vi "UHR-Fleezers Control (host) - Lorentz v3.vi"() -> ()   [LabVIEW 2014] (continued)
            n1765 = Number To Decimal String(number=w2676) -> (decimal integer string=w2678:string)  [unwired: 1 in]
            n1766 = Concatenate Strings("on, flow rate", w2678) -> (w2677:string)
            n1767 = Select(t=w2677, s=w2682, f="off") -> (s? t:f=w2686:string)
            n1768 = local read "Time (s)"() -> (w2680:dbl)
            n1769 = local read "log file ref"() -> (w2681:refnum<file>)
            n1770 = Concatenate Strings("pump 2 ", w2686) -> (w2684:string)
            n1771 = call "write to event log.vi"("log file ref"=w2681, "time"=w2680, "input string"=w2684) -> ()  [unwired: 8 in]
          }
        }
      }
      event "Sample Channel\nFlow": Value Change {
        n1772 = event-data() -> ()  [unwired: 7 out]
        n1773 = disable-structure shown="Disabled" {
          disable-tunnel: w2704 -> [w2711 _]
          frame Disabled {
            n1774 = Select(t="irun" ("string"), s="Sample Channel\nFlow", f="stop" ("string")) -> (s? t:f=w2706:string)
            n1775 = Concatenate Strings(w2706, "\r") -> (w2709:string)
            n1776 = VISA Write(VISA resource name=w2711, write buffer=w2709) -> ()  [unwired: 1 in, 3 out]
          }
          frame Enabled {
          }
        }
      }
      event "Start Flow": Value Change {
        n1777 = event-data() -> ()  [unwired: 7 out]
        n1778 = disable-structure shown="Disabled" {
          disable-tunnel: w2712 -> [w2713 _]
          frame Disabled {
            n1779 = local write "Sample Channel\nFlow"(TRUE ("Sample Channel\nFlow")) -> ()
            n1780 = local write "Start Flow"(FALSE ("Start Flow")) -> ()
            n1781 = Concatenate Strings("irun" ("string"), "\r") -> (w2717:string)
            n1782 = VISA Write(VISA resource name=w2713, write buffer=w2717) -> ()  [unwired: 1 in, 3 out]
          }
          frame Enabled {
          }
        }
      }
      event "Stop Flow": Value Change {
        n1783 = event-data() -> ()  [unwired: 7 out]
        n1784 = disable-structure shown="Disabled" {
          disable-tunnel: w2719 -> [w2721 _]
          frame Disabled {
            w2720 = FALSE ("Stop Flow")
            n1785 = local write "Stop Flow"(w2720) -> ()
            n1786 = local write "Sample Channel\nFlow"(w2720) -> ()
            n1787 = Concatenate Strings("stop" ("string"), "\r") -> (w2723:string)
            n1788 = VISA Write(VISA resource name=w2721, write buffer=w2723) -> ()  [unwired: 1 in, 3 out]
          }
          frame Enabled {
          }
        }
      }
      event "Flow rate (uL/h)": Value Change {
        n1789 = event-data() -> ()  [unwired: 7 out]
        n1790 = disable-structure shown="Disabled" {
          disable-tunnel: w2725 -> [w2727 _]
          frame Disabled {
            n1791 = Number To Decimal String(number="Flow rate (uL/h)") -> (decimal integer string=w2731:string)  [unwired: 1 in]
            n1792 = Concatenate Strings("irate  " ("string"), w2731, " u/h" ("string"), "\r") -> (w2730:string)
            n1793 = VISA Write(VISA resource name=w2727, write buffer=w2730) -> ()  [unwired: 1 in, 3 out]
          }
          frame Enabled {
          }
        }
      }
      event "Flush Sample": Value Change {
        n1794 = event-data() -> ()  [unwired: 7 out]
        n1795 = disable-structure shown="Disabled" {
          disable-tunnel: ["Flush Sample" _] -> w2734
          disable-tunnel: w2733 -> [w2740 _]
          frame Disabled {
            n1796 = flat-sequence {
              tunnel: w2740 -> [w2781]
              tunnel: [w2761] -> w2744
              tunnel: [w2757] -> w2743
              tunnel: ["Volume (uL)"] -> w2739
              tunnel: ["Flush rate (uL/m)"] -> w2738
              tunnel: w2744 -> [w2785]
              tunnel: [w2785] -> w2742
              tunnel: w2743 -> [w2784]
              tunnel: w2742 -> [w2790]
              frame #0 {
                # "set paramaters (rate, volume) for flush, clear volume"
                n1797 = Number To Decimal String(number="Flush rate (uL/m)") -> (decimal integer string=w2777:string)  [unwired: 1 in]
                n1798 = Concatenate Strings("irate  " ("string"), w2777, " u/m" ("string"), "\r") -> (w2779:string)
                n1799 = VISA Write(VISA resource name=w2781, write buffer=w2779) -> (VISA resource name out=w2775:refnum<visa-resource-name>)  [unwired: 1 in, 2 out]
                n1800 = Reciprocal(x="Flush rate (uL/m)") -> (1/x=w2760:dbl)
                n1801 = Number To Decimal String(number="Volume (uL)") -> (decimal integer string=w2766:string)  [unwired: 1 in]
                n1802 = Multiply(x="Volume (uL)", y=w2760) -> (x*y=w2759:dbl)
                n1803 = Concatenate Strings("tvolume  " ("string"), w2766, " u" ("string"), "\r") -> (w2764:string)
                n1804 = Multiply(x=w2759, y=60000.0) -> (x*y=w2757:dbl)
                n1805 = VISA Write(VISA resource name=w2775, write buffer=w2764) -> (VISA resource name out=w2763:refnum<visa-resource-name>)  [unwired: 1 in, 2 out]
                n1806 = Concatenate Strings("cvolume" ("string"), "\r") -> (w2762:string)
                n1807 = VISA Write(VISA resource name=w2763, write buffer=w2762) -> (VISA resource name out=w2773:refnum<visa-resource-name>)  [unwired: 1 in, 2 out]
                n1808 = Concatenate Strings("irun" ("string"), "\r") -> (w2771:string)
                n1809 = VISA Write(VISA resource name=w2773, write buffer=w2771) -> (VISA resource name out=w2761:refnum<visa-resource-name>)  [unwired: 1 in, 2 out]
              }
              frame #1 {
                # "Have to wait until\nflow is done to reset\nrate"
                n1810 = Add(x=w2784, y=100.0) -> (x+y=w2783:dbl)
                n1811 = Wait (ms)(milliseconds to wait=w2783) -> ()  [unwired: 1 out]
              }
              frame #2 {
                # "reset flow rate to usual flow rate"
                n1812 = local read "Flow rate (uL/h)"() -> (w2796:dbl)
                n1813 = Number To Decimal String(number=w2796) -> (decimal integer string=w2794:string)  [unwired: 1 in]
                n1814 = Concatenate Strings("irate  " ("string"), w2794, " u/h" ("string"), "\r") -> (w2792:string)
                n1815 = VISA Write(VISA resource name=w2790, write buffer=w2792) -> (VISA resource name out=w2786:refnum<visa-resource-name>)  [unwired: 1 in, 2 out]
                n1816 = Concatenate Strings("cvolume" ("string"), "\r") -> (w2787:string)
                n1817 = VISA Write(VISA resource name=w2786, write buffer=w2787) -> ()  [unwired: 1 in, 3 out]
              }
            }
            n1818 = local read "Save Event Log?"() -> (w2736:bool)
            n1819 = local read "Saving..."() -> (w2735:bool)
            n1820 = And(x=w2736, y=w2735) -> (x .and. y?=w2737:bool)
            n1821 = case shown="True" w2737 {
              tunnel: w2739 -> [_ w2746]
              tunnel: w2738 -> [_ w2745]
              frame False {
              }
              frame True {
                n1822 = Number To Decimal String(number=w2746) -> (decimal integer string=w2750:string)  [unwired: 1 in]
                n1823 = Number To Decimal String(number=w2745) -> (decimal integer string=w2752:string)  [unwired: 1 in]
                n1824 = local read "log file ref"() -> (w2747:refnum<file>)
                n1825 = local read "Time (s)"() -> (w2748:dbl)
                n1826 = Concatenate Strings("pump 2 flushing ", w2750, " uL at ", w2752, " ul/min") -> (w2754:string)
                n1827 = call "write to event log.vi"("log file ref"=w2747, "time"=w2748, "input string"=w2754) -> ()  [unwired: 8 in]
              }
            }
          }
          frame Enabled {
          }
        }
      }
      event "Flush Pump 3": Value Change {
        n1828 = event-data() -> ()  [unwired: 7 out]
        n1829 = disable-structure shown="Disabled" {
          disable-tunnel: ["Flush Pump 3" _] -> w2798
          disable-tunnel: w2797 -> [w2804 _]
          frame Disabled {
            n1830 = flat-sequence {
              tunnel: w2804 -> [w2819]
              tunnel: ["Flush rate (uL/m) P3"] -> w2800
              tunnel: ["Volume (uL) P3"] -> w2799
              frame #0 {
                # "set paramaters (rate, volume) for flush, clear volume"
                n1831 = Number To Decimal String(number="Flush rate (uL/m) P3") -> (decimal integer string=w2839:string)  [unwired: 1 in]
                n1832 = local write "Inject Pump 3"(TRUE ("Inject Pump 3")) -> ()
                n1833 = Concatenate Strings("irate  " ("string"), w2839, " u/m" ("string"), "\r") -> (w2841:string)
                n1834 = VISA Write(VISA resource name=w2819, write buffer=w2841) -> (VISA resource name out=w2837:refnum<visa-resource-name>)  [unwired: 1 in, 2 out]
                n1835 = Reciprocal(x="Flush rate (uL/m) P3") -> (1/x=w2823:dbl)
                n1836 = Number To Decimal String(number="Volume (uL) P3") -> (decimal integer string=w2828:string)  [unwired: 1 in]
                n1837 = Multiply(x="Volume (uL) P3", y=w2823) -> (x*y=w2822:dbl)
                n1838 = Concatenate Strings("tvolume  " ("string"), w2828, " u" ("string"), "\r") -> (w2826:string)
                n1839 = Multiply(x=w2822, y=60.0) -> (x*y=→"HP3 Flush Time (s)":dbl)
                n1840 = VISA Write(VISA resource name=w2837, write buffer=w2826) -> (VISA resource name out=w2825:refnum<visa-resource-name>)  [unwired: 1 in, 2 out]
                n1841 = Concatenate Strings("cvolume" ("string"), "\r") -> (w2824:string)
                n1842 = VISA Write(VISA resource name=w2825, write buffer=w2824) -> (VISA resource name out=w2835:refnum<visa-resource-name>)  [unwired: 1 in, 2 out]
                n1843 = Concatenate Strings("irun" ("string"), "\r") -> (w2833:string)
                n1844 = VISA Write(VISA resource name=w2835, write buffer=w2833) -> ()  [unwired: 1 in, 3 out]
              }
              frame #1 {
                "Flushing P3" <- TRUE ("Flushing P3")
              }
            }
            n1845 = local read "Save Event Log?"() -> (w2802:bool)
            n1846 = local read "Saving..."() -> (w2803:bool)
            n1847 = And(x=w2802, y=w2803) -> (x .and. y?=w2801:bool)
            n1848 = case shown="True" w2801 {
              tunnel: w2800 -> [_ w2807]
              tunnel: w2799 -> [_ w2806]
              frame False {
              }
              frame True {
                n1849 = Number To Decimal String(number=w2806) -> (decimal integer string=w2811:string)  [unwired: 1 in]
                n1850 = Number To Decimal String(number=w2807) -> (decimal integer string=w2813:string)  [unwired: 1 in]
                n1851 = local read "log file ref"() -> (w2808:refnum<file>)
                n1852 = local read "Time (s)"() -> (w2809:dbl)
                n1853 = Concatenate Strings("pump 3 flushing ", w2811, " uL at ", w2813, " ul/min") -> (w2815:string)
                n1854 = call "write to event log.vi"("log file ref"=w2808, "time"=w2809, "input string"=w2815) -> ()  [unwired: 8 in]
              }
            }
          }
          frame Enabled {
          }
        }
      }
      event "Flush Pump 1": Value Change {
        n1855 = event-data() -> ()  [unwired: 7 out]
        n1856 = disable-structure shown="Disabled" {
          disable-tunnel: ["Flush Pump 1" _] -> w2845
          disable-tunnel: w2844 -> [w2851 _]
          frame Disabled {
            n1857 = flat-sequence {
              tunnel: [w2872] -> w2853
              tunnel: w2851 -> [w2867]
              tunnel: ["Volume (uL) P1"] -> w2847
              tunnel: ["Flush rate (uL/m) P1"] -> w2846
              tunnel: w2853 -> [_]
              frame #0 {
                # "set paramaters (rate, volume) for flush, clear volume"
                n1858 = local write "Inject Pump 1"(TRUE ("Inject Pump 1")) -> ()
                n1859 = Number To Decimal String(number="Flush rate (uL/m) P1") -> (decimal integer string=w2888:string)  [unwired: 1 in]
                n1860 = Concatenate Strings("irate  " ("string"), w2888, " u/m" ("string"), "\r") -> (w2890:string)
                n1861 = VISA Write(VISA resource name=w2867, write buffer=w2890) -> (VISA resource name out=w2886:refnum<visa-resource-name>)  [unwired: 1 in, 2 out]
                n1862 = Reciprocal(x="Flush rate (uL/m) P1") -> (1/x=w2871:dbl)
                n1863 = Number To Decimal String(number="Volume (uL) P1") -> (decimal integer string=w2877:string)  [unwired: 1 in]
                n1864 = Multiply(x="Volume (uL) P1", y=w2871) -> (x*y=w2870:dbl)
                n1865 = Concatenate Strings("tvolume  " ("string"), w2877, " u" ("string"), "\r") -> (w2875:string)
                n1866 = Multiply(x=w2870, y=60.0) -> (x*y=→"HP1 Flush Time (s)":dbl)
                n1867 = VISA Write(VISA resource name=w2886, write buffer=w2875) -> (VISA resource name out=w2874:refnum<visa-resource-name>)  [unwired: 1 in, 2 out]
                n1868 = Concatenate Strings("cvolume" ("string"), "\r") -> (w2873:string)
                n1869 = VISA Write(VISA resource name=w2874, write buffer=w2873) -> (VISA resource name out=w2884:refnum<visa-resource-name>)  [unwired: 1 in, 2 out]
                n1870 = Concatenate Strings("irun" ("string"), "\r") -> (w2882:string)
                n1871 = VISA Write(VISA resource name=w2884, write buffer=w2882) -> (VISA resource name out=w2872:refnum<visa-resource-name>)  [unwired: 1 in, 2 out]
              }
              frame #1 {
                "Flushing P1" <- TRUE ("Flushing P3")
              }
            }
            n1872 = local read "Saving..."() -> (w2848:bool)
            n1873 = local read "Save Event Log?"() -> (w2849:bool)
            n1874 = And(x=w2849, y=w2848) -> (x .and. y?=w2850:bool)
            n1875 = case shown="True" w2850 {
              tunnel: w2847 -> [_ w2856]
              tunnel: w2846 -> [_ w2855]
              frame False {
              }
              frame True {
                n1876 = Number To Decimal String(number=w2856) -> (decimal integer string=w2860:string)  [unwired: 1 in]
                n1877 = Number To Decimal String(number=w2855) -> (decimal integer string=w2858:string)  [unwired: 1 in]
                n1878 = local read "log file ref"() -> (w2862:refnum<file>)
                n1879 = local read "Time (s)"() -> (w2863:dbl)
                n1880 = Concatenate Strings("pump 1 flushing ", w2860, " uL at ", w2858, " ul/min") -> (w2854:string)
                n1881 = call "write to event log.vi"("log file ref"=w2862, "time"=w2863, "input string"=w2854) -> ()  [unwired: 8 in]
              }
            }
          }
          frame Enabled {
          }
        }
      }
      event "Clear Volume": Value Change {
        n1882 = event-data() -> ()  [unwired: 7 out]
        n1883 = disable-structure shown="Disabled" {
          disable-tunnel: ["Clear Volume" _] -> w2894
          disable-tunnel: w2893 -> [w2895 _]
          frame Disabled {
            n1884 = Concatenate Strings("cvolume" ("string"), "\r") -> (w2896:string)
            n1885 = VISA Write(VISA resource name=w2895, write buffer=w2896) -> ()  [unwired: 1 in, 3 out]
          }
          frame Enabled {
          }
        }
      }
      event "Clear Volume P3": Value Change {
        n1886 = event-data() -> ()  [unwired: 7 out]
        n1887 = disable-structure shown="Disabled" {
          disable-tunnel: w2900 -> [w2902 _]
          frame Disabled {
            n1888 = Concatenate Strings("cvolume" ("string"), "\r") -> (w2903:string)
            n1889 = VISA Write(VISA resource name=w2902, write buffer=w2903) -> ()  [unwired: 1 in, 3 out]
            n1890 = local write "Clear Volume P3"(FALSE ("Clear Volume P3")) -> ()
          }
          frame Enabled {
          }
        }
      }
      event "Clear Volume P1": Value Change {
        n1891 = event-data() -> ()  [unwired: 7 out]
        n1892 = disable-structure shown="Disabled" {
          disable-tunnel: w2906 -> [w2908 _]
          frame Disabled {
            n1893 = Concatenate Strings("cvolume" ("string"), "\r") -> (w2909:string)
            n1894 = local write "Clear Volume P1"(FALSE ("Clear Volume P1")) -> ()
            n1895 = VISA Write(VISA resource name=w2908, write buffer=w2909) -> ()  [unwired: 1 in, 3 out]
          }
          frame Enabled {
          }
        }
      }
      event "Display On P3": Value Change {
        n1896 = event-data() -> ()  [unwired: 7 out]
        n1897 = disable-structure shown="Disabled" {
          disable-tunnel: w2912 -> [w2913 _]
          frame Disabled {
            n1898 = Select(t="dim 100", s="Display On P3", f="dim 0") -> (s? t:f=w2916:string)
            n1899 = Concatenate Strings(w2916, "\r") -> (w2918:string)
            n1900 = VISA Write(VISA resource name=w2913, write buffer=w2918) -> ()  [unwired: 1 in, 3 out]
          }
          frame Enabled {
          }
        }
      }
      event "Display On P1": Value Change {
        n1901 = event-data() -> ()  [unwired: 7 out]
        n1902 = disable-structure shown="Disabled" {
          disable-tunnel: w2920 -> [w2921 _]
          frame Disabled {
            n1903 = Select(t="dim 100", s="Display On P1", f="dim 0") -> (s? t:f=w2924:string)
            n1904 = Concatenate Strings(w2924, "\r") -> (w2926:string)
            n1905 = VISA Write(VISA resource name=w2921, write buffer=w2926) -> ()  [unwired: 1 in, 3 out]
          }
          frame Enabled {
          }
        }
      }
      event "Retract Pump 3": Value Change {
        n1906 = event-data() -> ()  [unwired: 7 out]
        n1907 = disable-structure shown="Disabled" {
          disable-tunnel: w2928 -> [w2929 _]
          frame Disabled {
            n1908 = local write "Retract Pump 3"(FALSE ("Retract Pump 3")) -> ()
            n1909 = case shown="True" "Retract Pump 3" {
              tunnel: w2929 -> [_ w2932]
              frame False {
              }
              frame True {
                n1910 = Number To Decimal String(number="Retract Rate (uL/m)") -> (decimal integer string=w2950:string)  [unwired: 1 in]
                n1911 = Concatenate Strings("wrate  " ("string"), w2950, " u/m" ("string"), "\r") -> (w2952:string)
                n1912 = VISA Write(VISA resource name=w2932, write buffer=w2952) -> (VISA resource name out=w2943:refnum<visa-resource-name>)  [unwired: 1 in, 2 out]
                n1913 = Number To Decimal String(number="Retract Vol 3 (uL)") -> (decimal integer string=w2945:string)  [unwired: 1 in]
                n1914 = Concatenate Strings("tvolume  " ("string"), w2945, " u" ("string"), "\r") -> (w2942:string)
                n1915 = VISA Write(VISA resource name=w2943, write buffer=w2942) -> (VISA resource name out=w2938:refnum<visa-resource-name>)  [unwired: 1 in, 2 out]
                n1916 = Concatenate Strings("cvolume" ("string"), "\r") -> (w2939:string)
                n1917 = VISA Write(VISA resource name=w2938, write buffer=w2939) -> (VISA resource name out=w2933:refnum<visa-resource-name>)  [unwired: 1 in, 2 out]
                n1918 = Concatenate Strings("wrun" ("string"), "\r") -> (w2934:string)
                n1919 = VISA Write(VISA resource name=w2933, write buffer=w2934) -> ()  [unwired: 1 in, 3 out]
              }
            }
          }
          frame Enabled {
          }
        }
      }
      event "Retract Pump 1": Value Change {
        n1920 = event-data() -> ()  [unwired: 7 out]
        n1921 = disable-structure shown="Disabled" {
          disable-tunnel: w2954 -> [w2955 _]
          frame Disabled {
            n1922 = local write "Retract Pump 1"(FALSE ("Retract Pump 1")) -> ()
            n1923 = case shown="True" "Retract Pump 1" {
              tunnel: w2955 -> [_ w2960]
              frame False {
              }
              frame True {
                n1924 = local read "Retract Rate (uL/m)"() -> (w2958:dbl)
                n1925 = Number To Decimal String(number=w2958) -> (decimal integer string=w2976:string)  [unwired: 1 in]
                n1926 = Concatenate Strings("wrate  " ("string"), w2976, " u/m" ("string"), "\r") -> (w2978:string)
                n1927 = VISA Write(VISA resource name=w2960, write buffer=w2978) -> (VISA resource name out=w2970:refnum<visa-resource-name>)  [unwired: 1 in, 2 out]
                n1928 = Number To Decimal String(number="Retract Vol 1 (uL)") -> (decimal integer string=w2972:string)  [unwired: 1 in]
                n1929 = Concatenate Strings("tvolume  " ("string"), w2972, " u" ("string"), "\r") -> (w2969:string)
                n1930 = VISA Write(VISA resource name=w2970, write buffer=w2969) -> (VISA resource name out=w2966:refnum<visa-resource-name>)  [unwired: 1 in, 2 out]
                n1931 = Concatenate Strings("cvolume" ("string"), "\r") -> (w2967:string)
                n1932 = VISA Write(VISA resource name=w2966, write buffer=w2967) -> (VISA resource name out=w2961:refnum<visa-resource-name>)  [unwired: 1 in, 2 out]
                n1933 = Concatenate Strings("wrun" ("string"), "\r") -> (w2962:string)
                n1934 = VISA Write(VISA resource name=w2961, write buffer=w2962) -> ()  [unwired: 1 in, 3 out]
              }
            }
          }
          frame Enabled {
          }
        }
      }
      event "Flip Green Filter": Value Change {
        n1935 = event-data() -> ()  [unwired: 7 out]
        n1936 = Not(x="Flip Green Filter") -> (.not. x?=w2981:bool)
        n1937 = local write "Flip Green Filter"(w2981) -> ()
        n1938 = flat-sequence {
          tunnel: [w2990] -> w2986
          tunnel: [w2989] -> w2985
          tunnel: w2980 -> [w2988]
          tunnel: [w2993] -> w2984
          tunnel: w2986 -> [w2993]
          tunnel: [w2992] -> w2983
          tunnel: w2985 -> [w2992]
          tunnel: w2984 -> [w2997]
          tunnel: w2983 -> [w2996]
          tunnel: [w2995] -> w2987
          frame #0 {
            n1939 = xnode "Read/Write Control"("FPGA VI Reference In"=w2988, "Green Filter Flipper"=TRUE) -> ("FPGA VI Reference Out"=w2990:T36, "error out"=w2989:errorcluster)  [unwired: 1 in]
          }
          frame #1 {
            n1940 = Wait (ms)(milliseconds to wait=u32 100) -> ()  [unwired: 1 out]
          }
          frame #2 {
            n1941 = xnode "Read/Write Control"("FPGA VI Reference In"=w2997, "error in"=w2996, "Green Filter Flipper"=FALSE) -> ("error out"=w2995:errorcluster)  [unwired: 1 out]
          }
        }
      }
      event "Pump 1 contents", "Pump 3 contents": Value Change {
        n1942 = event-data() -> ()  [unwired: 7 out]
        n1943 = local read "Pump 1 contents"() -> (→"Pump 1 cont disp":string)
        n1944 = local read "Pump 3 contents"() -> (→"Pump 3 cont disp":string)
      }
      event "Reset Trap Pos. FB": Value Change {
        n1945 = event-data() -> ()  [unwired: 7 out]
        n1946 = xnode "Read/Write Control"("FPGA VI Reference In"=w3001, "Trap Pos. FB Reset"="Reset Trap Pos. FB") -> ()  [unwired: 1 in, 2 out]
      }
      event "Rem fb disp offset": Value Change {
        n1947 = event-data() -> ()  [unwired: 7 out]
        n1948 = local write "Rem fb disp offset"(FALSE ("Rem fb disp offset")) -> ()
        n1949 = local read "Mean Trap Positions (nm)"() -> (w3004:T4)
        n1950 = local read "FB Trap Pos Offset"() -> (w3006:dbl)
        n1951 = Unbundle By Name(w3004) -> ("T1 X"=w3003:dbl)
        n1952 = Subtract(x=w3006, y=w3003) -> (x-y=w3005:dbl)
        n1953 = local write "FB Trap Pos Offset"(w3005) -> ()
      }
      event "Threshold (nm)": Value Change {
        n1954 = event-data() -> ()  [unwired: 7 out]
        n1955 = flat-sequence {
          tunnel: [w3011] -> w3009
          tunnel: w3008 -> [w3010]
          tunnel: w3009 -> [w3022]
          frame #0 {
            n1956 = xnode "Read/Write Control"("FPGA VI Reference In"=w3010) -> ("FPGA VI Reference Out"=w3014:T36, "error out"=w3013:errorcluster, "FPGA TTrig Thresh"=w3015:i64)  [unwired: 1 in]
            n1957 = local read "Threshold stored (nm)"() -> (w3021:dbl)
            n1958 = local read "Threshold (nm)"() -> (w3011:dbl)
            n1959 = local read "AOM X Cal (nm/MHz)"() -> (w3019:dbl)
            n1960 = Subtract(x=w3011, y=w3021) -> (x-y=w3020:dbl)
            n1961 = Divide(x=w3020, y=w3019) -> (x/y=w3017:dbl)
            n1962 = call "IR AOM freq to word.vi"("Frequency In (MHz)"=w3017) -> ("Frequency Word Out (double)"=w3018:dbl)
            n1963 = To Quad Integer(1:w3018) -> (0:w3016:i64)
            n1964 = Add(x=w3015, y=w3016) -> (x+y=w3012:i64)
            n1965 = xnode "Read/Write Control"("FPGA VI Reference In"=w3014, "error in"=w3013, "FPGA TTrig Thresh"=w3012) -> ()  [unwired: 2 out]
          }
          frame #1 {
            "Threshold stored (nm)" <- w3022
          }
        }
      }
      event "FB Trig Integrate": Value Change {
        n1966 = event-data() -> ()  [unwired: 7 out]
        n1967 = local read "FB Trig Integrate"() -> (w3025:u32)
        n1968 = xnode "Read/Write Control"("FPGA VI Reference In"=w3023, "FB Trig Integrate"=w3025) -> ("error out"=w3024:errorcluster)  [unwired: 1 in, 1 out]
      }
      event "11": Value Change {
        n1969 = event-data() -> ()  [unwired: 7 out]
        n1970 = local read "11"() -> (w3026:bool)
        n1971 = case shown="True" w3026 {
          frame False {
          }
          frame True {
            n1972 = local read "Messages"() -> (w3028:string)
            n1973 = call "Update messages.vi"("Message to add"="You kicked it up to 11!", "Old message string"=w3028) -> ("New message string"=w3029:string)
            n1974 = call <vilib>:"Beep.vi"() -> ()  [unwired: 12 in]
            n1975 = local write "Messages"(w3029) -> ()
          }
        }
      }
      event "Trap Pos. FB ON": Value Change {
        w3036 = 6.0  # clock mult.
        w3035 = 49152000.0  # TCXO frequ.
        n1976 = event-data() -> ()  [unwired: 7 out]
        n1977 = xnode "Read/Write Control"("FPGA VI Reference In"=w3030) -> ("FPGA VI Reference Out"=w3032:T36, "BD1 Frequency Out 1"=w3033:u64)  [unwired: 1 in, 1 out]
        n1978 = To Double Precision Float(number=w3033) -> (double precision float=w3037:dbl)
        n1979 = Multiply(x=w3035, y=w3036) -> (x*y=w3038:dbl)
        n1980 = Multiply(x=w3037, y=w3038) -> (x*y=w3039:dbl)
        n1981 = Scale By Power Of 2(n=-48, x=w3039) -> (x*2^n=w3041:dbl)
        n1982 = Divide(x=w3041, y=1000000.0) -> (x/y=w3034:dbl)
        n1983 = flat-sequence {
          tunnel: w3032 -> [w3047]
          tunnel: [w3046] -> w3043
          tunnel: "Trap Pos. FB ON" -> [w3045]
          tunnel: w3033 -> [w3044]
          tunnel: w3043 -> [w3053]
          tunnel: "Trap Pos. FB ON" -> [w3052]
          tunnel: w3034 -> [w3055]
          tunnel: "Trap Pos. FB ON" -> [w3054]
          frame #0 {
            n1984 = case shown="False" w3045 {
              tunnel: w3047 -> [w3049 w3051]
              tunnel: [w3050 w3051] -> w3046
              tunnel: w3044 -> [w3048 _]
              frame False {
                n1985 = xnode "Read/Write Control"("FPGA VI Reference In"=w3049, "BD 1 Frequency 1"=w3048) -> ("FPGA VI Reference Out"=w3050:T36)  [unwired: 1 in, 1 out]
              }
              frame True {
              }
            }
          }
          frame #1 {
            n1986 = xnode "Read/Write Control"("FPGA VI Reference In"=w3053, "Force feedback"=w3052) -> ()  [unwired: 1 in, 2 out]
          }
          frame #2 {
            n1987 = case shown="False" w3054 {
              tunnel: w3055 -> [w3056 _]
              frame False {
                n1988 = property on="BD 1 Frequency 1 (MHz)" class="DigNum (strict)"("Val(Sgnl)"=w3056) -> ()  [unwired: 2 in, 2 out]
              }
              frame True {
              }
            }
          }
        }
      }
      event "Remove Action Offset": Value Change {
        n1989 = event-data() -> ()  [unwired: 7 out]
        n1990 = local write "Remove Action Offset"(FALSE ("Remove Action Offset")) -> ()
        n1991 = local read "Trap Pos. FB Mult Factor"() -> (w3062:i64)
        n1992 = local read "Trap Pos FB Action"() -> (w3060:i64)
        n1993 = local read "Trap Pos. FB Offset Factor"() -> (w3058:i64)
        n1994 = Multiply(x=w3062, y=w3060) -> (x*y=w3061:i64)
        n1995 = Add(x=w3061, y=w3058) -> (x+y=w3059:i64)
        n1996 = local write "Trap Pos. FB Offset Factor"(w3059) -> ()
        n1997 = xnode "Read/Write Control"("FPGA VI Reference In"=w3057, "Trap Pos. FB Offset Factor"=w3059) -> ()  [unwired: 1 in, 2 out]
      }
      event "Remove Unwinding Offset": Value Change {
        n1998 = event-data() -> ()  [unwired: 7 out]
        n1999 = local write "Remove Unwinding Offset"(FALSE ("Remove Action Offset")) -> ()
        n2000 = local read "Trap Pos. FB Mult Factor"() -> (w3076:i64)
        n2001 = local read "Trap Pos FB Action"() -> (w3074:i64)
        n2002 = local read "Trap Pos. FB Offset Factor"() -> (w3073:i64)
        n2003 = Multiply(x=w3076, y=w3074) -> (x*y=w3075:i64)
        n2004 = local read "Trap Pos. FB Mult Factor"() -> (w3072:i64)
        n2005 = Add(x=w3075, y=w3073) -> (x+y=w3066:i64)
        n2006 = Multiply(x=32768, y="factor") -> (x*y=w3069:dbl)
        n2007 = Multiply(x=w3069, y=w3072) -> (x*y=w3071:dbl)
        n2008 = Subtract(x=w3066, y=w3071) -> (x-y=w3070:dbl)
        n2009 = To Quad Integer(1:w3070) -> (0:w3065:i64)
        n2010 = xnode "Read/Write Control"("FPGA VI Reference In"=w3064, "Trap Pos. FB Offset Factor"=w3065) -> ()  [unwired: 1 in, 2 out]
        n2011 = local write "Trap Pos. FB Offset Factor"(w3065) -> ()
      }
      event "Trap Pos. FB Range", "Trap Pos. FB Gains", "Trap Pos. FB Mult Factor", "Trap Pos. FB Offset Factor", "Trap Pos FB Negate Action", "Trap Pos FB Monitor\nT1 or T2", "Differential FB?", "Negate Diff?": Value Change {
        n2012 = event-data() -> ()  [unwired: 7 out]
        n2013 = local read "Negate Diff?"() -> (w3081:bool)
        n2014 = xnode "Read/Write Control"("FPGA VI Reference In"=w3080, "Trap Pos. FB Gains"="Trap Pos. FB Gains", "Trap pos. FB Range"="Trap Pos. FB Range", "Trap Pos. FB Mult Factor"="Trap Pos. FB Mult Factor", "Trap Pos. FB Offset Factor"="Trap Pos. FB Offset Factor", "Trap Pos FB Negate Action"="Trap Pos FB Negate Action", "Trap Pos FB Monitor T1 or T2"="Trap Pos FB Monitor\nT1 or T2", "AI1 X Scale"="Trap Pos. AI1 X Pre-scale", "Negate Diff?"=w3081, "Diff FB Measurement?"="Differential FB?") -> ()  [unwired: 1 in, 2 out]
      }
      event "Trap Pos FB SP", "Trap Pos FB SP 2", "Use SP 2": Value Change {
        n2015 = event-data() -> ()  [unwired: 7 out]
        n2016 = Select(t="Trap Pos FB SP 2", s="Use SP 2", f="Trap Pos FB SP") -> (s? t:f=w3089:fxp<+/-,16,1>)
        n2017 = xnode "Read/Write Control"("FPGA VI Reference In"=w3088, "Trap Pos. FB SP"=w3089) -> ()  [unwired: 1 in, 2 out]
      }
      event "Offset SP2 from SP1": Value Change {
        n2018 = event-data() -> ()  [unwired: 7 out]
        n2019 = local read "Trap Pos FB SP"() -> (w3095:fxp<+/-,16,1>)
        n2020 = Add(x=w3095, y="SP2 Offset") -> (x+y=w3093:fxp<+/-,16,1>)
        n2021 = property on="Trap Pos FB SP 2" class="DigNum (strict)"("Val(Sgnl)"=w3093) -> ()  [unwired: 2 in, 2 out]
        n2022 = local write "Offset SP2 from SP1"(FALSE ("Offset SP2 from SP1")) -> ()
      }
      event "Set Reading to\nSetpoint": Value Change {
        # "This is the actual PID input signal"
        n2023 = event-data() -> ()  [unwired: 7 out]
        n2024 = local write "Set Reading to\nSetpoint"(FALSE ("Set SP to Reading")) -> ()
        n2025 = xnode "Read/Write Control"("FPGA VI Reference In"=w3099) -> ("FPGA VI Reference Out"=w3102:T36, "error out"=w3101:errorcluster, "Trap Pos FB Int-Norm Signal"=w3100:fxp<+/-,16,1>, "BD1 Frequency Out 1"=w3098:u64)  [unwired: 1 in]
        n2026 = local read "Differential FB?"() -> (w3103:bool)
        n2027 = case shown="False" w3103 {
          tunnel: [w3132 w3139] -> w3097
          tunnel: w3100 -> [w3130 w3139]
          frame False {
            n2028 = local read "Trap Pos FB Monitor\nT1 or T2"() -> (w3135:bool)
            n2029 = local read "Trap X AI1 (DMA)"() -> (w3138:T19)
            n2030 = Unbundle By Name(w3138) -> ("Set 1"=w3137:fxp<+/-,16,1>, "Set 2"=w3136:fxp<+/-,16,1>)
            n2031 = Select(t=w3137, s=w3135, f=w3136) -> (s? t:f=w3134:fxp<+/-,16,1>)
            n2032 = Not(x="Set SP Using...") -> (.not. x?=w3131:bool)
            n2033 = Select(t=w3130, s=w3131, f=w3134) -> (s? t:f=w3132:fxp<+/-,16,1>)
          }
          frame True {
          }
        }
        n2034 = disable-structure shown="Disabled" {
          disable-tunnel: _ -> [w3108 _]
          disable-tunnel: w3098 -> [w3107 _]
          disable-tunnel: w3097 -> [w3106 _]
          frame Disabled {
            n2035 = case shown="True" w3108 {
              tunnel: [w3109 w3111] -> w3105
              tunnel: w3106 -> [w3109 w3110]
              tunnel: w3107 -> [_ w3129]
              frame False {
              }
              frame True {
                w3127 = 6.0  # clock mult.
                w3128 = 49152000.0  # TCXO frequ.
                # "Added by Ronen - for the real time\nchange of the setpoint to accomodate \nchanges in the offset."
                n2036 = To Double Precision Float(number=w3129) -> (double precision float=w3126:dbl)
                n2037 = local read "BD 1 Frequency 2 (MHz)"() -> (w3119:dbl)
                n2038 = Multiply(x=w3128, y=w3127) -> (x*y=w3125:dbl)
                n2039 = Multiply(x=w3126, y=w3125) -> (x*y=w3124:dbl)
                n2040 = local read "Offset file step size"() -> (w3117:dbl)
                n2041 = Scale By Power Of 2(n=-48, x=w3124) -> (x*2^n=w3122:dbl)
                n2042 = Divide(x=w3122, y=1000000.0) -> (x/y=w3120:dbl)
                n2043 = Subtract(x=w3119, y=w3120) -> (x-y=w3118:dbl)
                n2044 = Divide(x=w3118, y=w3117) -> (x/y=w3116:dbl)
                n2045 = local read item#-1() -> (w3114)
                n2046 = To Long Integer(number=w3116) -> (32bit integer=w3115:i32)
                n2047 = Index Array(array=w3114, index=w3115) -> (element=w3113)
                n2048 = To Fixed-Point(number=w3113) -> (fixed-point=w3112:fxp<+/-,16,1>)  [unwired: 1 in]
                n2049 = Add(x=w3110, y=w3112) -> (x+y=w3111:fxp<+/-,17,2>)
              }
            }
            "Offset corrected setpoint" <- w3105
          }
          frame Enabled {
          }
        }
        n2050 = local write "Trap Pos FB SP"(w3097) -> ()
        n2051 = xnode "Read/Write Control"("FPGA VI Reference In"=w3102, "error in"=w3101, "Trap Pos. FB SP"=w3097) -> ()  [unwired: 2 out]
      }
      event "Trap Pos. FB Out Scale 2^n": Value Change {
        n2052 = event-data() -> ()  [unwired: 7 out]
        n2053 = Scale By Power Of 2(n="Trap Pos. FB Out Scale 2^n", x=ext 1.0) -> (x*2^n=w3140:ext)
        n2054 = property on="Trap Pos. FB Mult Factor" class="DigNum (strict)"("Val(Sgnl)"=w3140) -> ()  [unwired: 2 in, 2 out]
      }
      event "Trap Pos FB Int Count": Value Change {
        n2055 = event-data() -> ()  [unwired: 7 out]
        n2056 = xnode "Read/Write Control"("FPGA VI Reference In"=w3143, "Trap Pos FB Int Count"="Trap Pos FB Int Count") -> ()  [unwired: 1 in, 2 out]
      }
      event "Display Saved Data": Value Change {
        n2057 = event-data() -> ()  [unwired: 7 out]
        n2058 = case shown="\"Amp Current\"" "Display Saved Data" {
          frame "Bead Seperation", Default {
            n2059 = property on="Amp current" class="WFGraph (strict)"("Visible"=FALSE) -> ()  [unwired: 2 in, 2 out]
            n2060 = property on="Trap Delta Graph" class="WFGraph (strict)"("Visible"=TRUE) -> ()  [unwired: 2 in, 2 out]
            n2061 = property on="Saved trap pos" class="WFGraph (strict)"("Visible"=FALSE) -> ()  [unwired: 2 in, 2 out]
          }
          frame "Amp Current" {
            n2062 = property on="Saved trap pos" class="WFGraph (strict)"("Visible"=FALSE) -> ()  [unwired: 2 in, 2 out]
            n2063 = property on="Trap Delta Graph" class="WFGraph (strict)"("Visible"=FALSE) -> ()  [unwired: 2 in, 2 out]
            n2064 = property on="Amp current" class="WFGraph (strict)"("Visible"=TRUE) -> ()  [unwired: 2 in, 2 out]
          }
          frame "Trap Position" {
            n2065 = property on="Saved trap pos" class="WFGraph (strict)"("Visible"=TRUE) -> ()  [unwired: 2 in, 2 out]
            n2066 = property on="Trap Delta Graph" class="WFGraph (strict)"("Visible"=FALSE) -> ()  [unwired: 2 in, 2 out]
            n2067 = property on="Amp current" class="WFGraph (strict)"("Visible"=FALSE) -> ()  [unwired: 2 in, 2 out]
          }
        }
      }
      event "Calibration": Value Change {
        n2068 = event-data() -> ()  [unwired: 7 out]
        n2069 = local read "X or Y?"() -> (w3171:bool)
        n2070 = local read "Calibration"() -> (w3168:u16)
        n2071 = Select(t="X" ("Label.Text"), s=w3171, f="Y" ("Label.Text")) -> (s? t:f=w3165:string)
        n2072 = case shown="0, Default" w3168 {
          tunnel: ["Position (V)" ("Label.Text") "Position (nm)" ("Label.Text") "Force (pN)" ("Label.Text")] -> w3162
          tunnel: [" (V)" ("Label.Text") " (nm)" ("Label.Text") " (pN)" ("Label.Text")] -> w3159
          frame 0, Default {
          }
          frame 1 {
          }
          frame 2 {
          }
        }
        n2073 = Concatenate Strings("T1 " ("Label.Text"), w3165) -> (w3161:string)
        n2074 = Concatenate Strings("T2 " ("Label.Text"), w3165) -> (w3160:string)
        n2075 = property on="Force" class="WFChart (strict)"("YScale.NameLbl.Text"=w3162) -> ()  [unwired: 2 in, 2 out]
        n2076 = Concatenate Strings("Mean" ("Label.Text"), w3159) -> (w3158:string)
        n2077 = Concatenate Strings(w3161, w3159) -> (w3157:string)
        n2078 = Concatenate Strings(w3160, w3159) -> (w3156:string)
        n2079 = Concatenate Strings("Difference" ("Label.Text"), w3159) -> (w3155:string)
        n2080 = property on="Mean" class="DigNum (strict)"("Caption.Text"=w3158) -> ()  [unwired: 2 in, 2 out]
        n2081 = property on="T1 X" class="DigNum (strict)"("Caption.Text"=w3157) -> ()  [unwired: 2 in, 2 out]
        n2082 = property on="T2 X" class="DigNum (strict)"("Caption.Text"=w3156) -> ()  [unwired: 2 in, 2 out]
        n2083 = property on="Difference" class="DigNum (strict)"("Caption.Text"=w3155) -> ()  [unwired: 2 in, 2 out]
      }
      event "Base N trap periods", "Period scale factor", "Trap osc amp (MHz)", "Cal sets to save", "# Samples/trap", "Total Counts (ticks)": Value Change {
        w3178 = 1.0
        w3184 = u32 0 ("y")
        # "scales 0 to 2pi"
        # "Create vector of trap offset (oscillation) values."
        # "Compute oscillation period as a multiple of the trap period. Should also fit nicely as a factor of the DMA period.\nCompare ticks for accurate commensurability check."
        # "Oscillation frequency needs to be commensurate\nwith the data save time."
        # "Be commensurate with total save time/100 (or so). That way you are guaranteed you can average spectra at least 100x."
        n2084 = event-data() -> ()  [unwired: 7 out]
        n2085 = local read "Total Counts (ticks)"() -> (w3200:u16)
        n2086 = To Unsigned Long Integer(number=w3200) -> (unsigned 32bit integer=w3210:u32)
        n2087 = Multiply "Base osc period (ticks)"(x=w3210, y="Base N trap periods") -> (x*y=w3201:u32)
        n2088 = local read "# Samples/trap"() -> (w3205:u32)
        n2089 = Multiply "Scaled osc period (ticks)"(x=w3201, y="Period scale factor") -> (x*y=w3202:dbl)
        n2090 = Multiply(x="Base N trap periods", y="Period scale factor") -> ()  [unwired: 1 out]
        n2091 = local read "Cal sets to save"() -> (w3206:u32)
        n2092 = To Unsigned Quad Integer(1:w3202) -> (0:w3192:u64)
        n2093 = for "vector 0 to N -1" {
          N: w3178 -> [_]
          tunnel: [w3227] -> w3198 mode=indexing
          i -> [w3227]
        }
        n2094 = Multiply "Ticks/DMA"(x=w3205, y=w3210) -> (x*y=w3209:u32)
        n2095 = Multiply "Scaled osc period (s)"(x=w3192, y=2.5e-08) -> (x*y=w3204:dbl)
        "Trap OSC Period (s)" <- w3204
        n2096 = Reciprocal(x=w3204) -> (1/x=→"A cal freq (Hz)":dbl)
        n2097 = Multiply(x=w3198, y=6.283185307179586) -> (x*y=w3213:dbl[])
        n2098 = Quotient & Remainder(x=w3209, y=w3192) -> (x-y*floor(x/y)=w3185:u64, floor(x/y)=→"N osc / DMA":u64)
        "DMA remainder" <- w3185
        n2099 = Multiply "Total trap ticks"(x=w3206, y=w3209) -> (x*y=w3193:u32)
        n2100 = Divide(x=w3213, y=w3178) -> (x/y=w3214:dbl[])
        n2101 = Sine(x=w3214) -> (sin(x)=w3215:dbl[])
        n2102 = Quotient & Remainder(x=w3193, y=100) -> (x-y*floor(x/y)=w3188:u32, floor(x/y)=w3208:u32)
        "Total save/100 remainder" <- w3188
        n2103 = Multiply "Single period osc vector"(x=w3215, y="Trap osc amp (MHz)") -> (x*y=w3191:dbl[])
        n2104 = Quotient & Remainder(x=w3208, y=w3192) -> (x-y*floor(x/y)=w3187:u64, floor(x/y)=→"N osc/ (total save/100)":u64)
        "(total save/100) /osc period remainder" <- w3187
        n2105 = Quotient & Remainder(x=w3193, y=w3192) -> (x-y*floor(x/y)=w3186:u64)  [unwired: 1 out]
        "N trap osc periods per save remainder" <- w3186
        n2106 = call "IR AOM freq to word - vec.vi"("Frequency In (double vec, MHz)"=w3191) -> ("Frequency Word Out"=w3190:dbl[])
        n2107 = To Quad Integer(1:w3190) -> (0:w3189:i64[])
        n2108 = disable-structure shown="Disabled" {
          disable-tunnel: w3197 -> [w3219 _]
          disable-tunnel: w3189 -> [w3217 _]
          frame Disabled {
            n2109 = xnode "Read/Write Control"("FPGA VI Reference In"=w3219) -> ("FPGA VI Reference Out"=w3218:T36)  [unwired: 3 in, 1 out]
            n2110 = flat-sequence {
              tunnel: w3217 -> [w3222]
              tunnel: w3218 -> [w3221]
              frame #0 {
                n2111 = for "Write data to fpga memory" {
                  tunnel: w3221 -> [w3224]
                  tunnel: w3222 -> [_] mode=indexing
                  (unwired) TRUE ("Ready Write")
                  n2112 = xnode "Read/Write Control"("FPGA VI Reference In"=w3224) -> ("FPGA VI Reference Out"=w3223:T36)  [unwired: 4 in, 1 out]
                  n2113 = while {
                    tunnel: w3223 -> [w3225]
                    stop <- _ continue-if-true
                    n2114 = xnode "Read/Write Control"("FPGA VI Reference In"=w3225) -> ()  [unwired: 1 in, 3 out]
                  }
                }
                "Writing waveform to fpga memory" <- TRUE ("Writing waveform to fpga memory")
              }
              frame #1 {
                n2115 = local write "Writing waveform to fpga memory"(FALSE ("Writing waveform to fpga memory")) -> ()
              }
            }
          }
          frame Enabled {
          }
        }
        n2116 = Equal?(x=w3187, y=w3184) -> (x = y?=w3182:bool)
        n2117 = Equal?(x=w3188, y=w3184) -> (x = y?=w3183:bool)
        n2118 = Equal?(x=w3185, y=w3184) -> (x = y?=w3180:bool)
        n2119 = Equal?(x=w3186, y=w3184) -> (x = y?=w3181:bool)
        n2120 = Compound Arithmetic op=AND(w3183, w3182, w3181, w3180) -> (→"Good freq?":bool)
      }
      event "Osc trap cont.", "Osc traps", "T1 Osc Enable", "T2 Osc Enable": Value Change {
        n2121 = event-data() -> ()  [unwired: 7 out]
        n2122 = disable-structure shown="Disabled" {
          disable-tunnel: w3228 -> [w3231 _]
          frame Disabled {
            n2123 = xnode "Read/Write Control"("FPGA VI Reference In"=w3231, "Trap 1 osc enable"="T1 Osc Enable", "Trap 2 osc enable"="T2 Osc Enable") -> ()  [unwired: 1 in, 2 out]
          }
          frame Enabled {
          }
        }
      }
      event "Pressure Pump Voltage (+/-10V)": Value Change {
        n2124 = event-data() -> ()  [unwired: 7 out]
        n2125 = disable-structure shown="Disabled" {
          disable-tunnel: w3232 -> [w3236 _]
          frame Disabled {
            n2126 = Divide(x="Pressure Pump Voltage (+/-10V)", y=10.0) -> (x/y=w3233:dbl)
            n2127 = Multiply(x=w3233, y=32767.0) -> (x*y=w3234:dbl)
            n2128 = xnode "Read/Write Control"("FPGA VI Reference In"=w3236, "Pressure Pump"=w3234) -> ()  [unwired: 1 in, 2 out]
          }
          frame Enabled {
          }
        }
      }
      event "Dynamic Force FB (ronen)": Value Change {
        # "Added by ronen - for feedback on trap position by changing the actual frequency and not the set frequency - for increasing the range of feedback."
        n2129 = event-data() -> ()  [unwired: 7 out]
        n2130 = xnode "Read/Write Control"("FPGA VI Reference In"=w3240, "Dynamic Force FB (Ronen)"="Dynamic Force FB (ronen)") -> ()  [unwired: 1 in, 2 out]
      }
      event "Read Setpoint Correction File": Value Change {
        n2131 = event-data() -> ()  [unwired: 7 out]
        n2132 = local write "Read Setpoint Correction File"(FALSE ("Read Setpoint Correction File")) -> ()
        n2133 = Open/Create/Replace File(file path (use dialog)="Setpoint Correction Offset File", operation (0:open)=T44."open", access (0:read/write)=enum16{"read/write", "read-only", "write-only"}."read-only") -> (refnum out=w3264:refnum<file>)  [unwired: 1 in, 4 out]
        n2134 = Deny Access(7:w3264) -> (3:w3263:refnum<file>)  [unwired: 1 in, 2 out]
        n2135 = Read from Binary File(5:0.0, 9:T45."big-endian, network order" ("byte order (0:big-endian, network order)"), 10:-1 ("count (1)"), 11:w3263) -> (2:w3257:dbl[], 3:w3262:refnum<file>)  [unwired: 1 in, 3 out]
        n2136 = Close File(refnum=w3262) -> ()  [unwired: 1 in, 2 out]
        n2137 = Array Subset(array=w3257, index=3) -> (w3258:dbl[])  [unwired: 1 in]
        n2138 = Index Array(array=w3257, index=0) -> (element=w3246:dbl)
        n2139 = local read "T2 calibration"() -> (w3245:T8)
        n2140 = local read "T1 calibration"() -> (w3253:T9)
        n2141 = local write "Offset file step size"(w3246) -> ()
        n2142 = Unbundle By Name(w3245) -> ("T2 alpha_x (nm/V)"=w3248:dbl, "T2 kappa_x (pN/nm)"=w3247:dbl)
        n2143 = Unbundle By Name(w3253) -> ("T1 alpha_x (nm/V)"=w3250:dbl, "T1 kappa_x (pN/nm)"=w3249:dbl)
        n2144 = Multiply(x=w3250, y=w3249) -> (x*y=w3251:dbl)
        n2145 = Multiply(x=w3248, y=w3247) -> (x*y=w3252:dbl)
        n2146 = Decimate 1D Array(w3258) -> (w3255:dbl[], w3254:dbl[])  [unwired: 1 out]
        n2147 = Divide(x=w3252, y=w3251) -> (x/y=w3242:dbl)
        n2148 = property on="B factor" class="DigNum (strict)"("Val(Sgnl)"=w3242) -> ()  [unwired: 2 in, 2 out]
        n2149 = Multiply(x=w3254, y=w3242) -> (x*y=w3256:dbl[])
        n2150 = Subtract(x=w3255, y=w3256) -> (x-y=w3241:dbl[])
        n2151 = local read "Offset Values"() -> (w3244:T20)
        n2152 = Bundle By Name(cluster=w3244, "Trap 1X offset"=w3255, "Trap 2X offset"=w3254) -> (w3243:T20)
        n2153 = local write "Offset Values"(w3243) -> ()
        n2154 = property on="Setpoint offset\ncorrection values" class="Arr (strict)"("Val(Sgnl)"=w3241) -> ()  [unwired: 2 in, 2 out]
      }
      event "B factor", "Setpoint offset\ncorrection values", "Target Force (pN)": Value Change {
        w3301 = 6.0  # clock mult.
        w3302 = 49152000.0  # TCXO frequ.
        n2155 = event-data() -> ()  [unwired: 7 out]
        n2156 = local read "B factor"() -> (w3303:dbl)
        n2157 = xnode "Read/Write Control"("FPGA VI Reference In"=w3304, "B factor"=w3303) -> ("BD1 Frequency Out 1"=w3294:u64)  [unwired: 1 in, 2 out]
        n2158 = To Double Precision Float(number=w3294) -> (double precision float=w3300:dbl)
        n2159 = local read "BD 1 Frequency 2 (MHz)"() -> (w3292:dbl)
        n2160 = Multiply(x=w3302, y=w3301) -> (x*y=w3299:dbl)
        n2161 = Multiply(x=w3300, y=w3299) -> (x*y=w3298:dbl)
        n2162 = Scale By Power Of 2(n=-48, x=w3298) -> (x*2^n=w3296:dbl)
        n2163 = Divide(x=w3296, y=1000000.0) -> (x/y=w3293:dbl)
        n2164 = Subtract(x=w3292, y=w3293) -> (x-y=w3280:dbl)
        n2165 = local read "Target Force (pN)"() -> (w3291:dbl)
        n2166 = local read "T1 calibration"() -> (w3289:T9)
        n2167 = local read "Offset file step size"() -> (w3279:dbl)
        n2168 = local read "Setpoint offset\ncorrection values"() -> (w3276:dbl[])
        n2169 = Unbundle By Name(w3289) -> ("T1 alpha_x (nm/V)"=w3288:dbl, "T1 kappa_x (pN/nm)"=w3287:dbl)
        n2170 = Multiply(x=w3291, y=2.0) -> (x*y=w3285:dbl)
        n2171 = Divide(x=w3280, y=w3279) -> (x/y=w3278:dbl)
        n2172 = local read "Negate Diff?"() -> (w3282:bool)
        n2173 = To Long Integer(number=w3278) -> (32bit integer=w3277:i32)
        n2174 = Multiply(x=w3288, y=w3287) -> (x*y=w3286:dbl)
        n2175 = Index Array(array=w3276, index=w3277) -> (element=w3274:dbl)
        n2176 = Divide(x=w3285, y=w3286) -> (x/y=w3281:dbl)
        n2177 = Select(t=1, s=w3282, f=-1) -> (s? t:f=w3275:i32)
        n2178 = Multiply(x=w3275, y=w3274) -> (x*y=w3273:dbl)
        n2179 = Add(x=w3281, y=w3273) -> (x+y=w3272:dbl)
        n2180 = To Fixed-Point(number=w3272) -> (fixed-point=w3271:fxp<+/-,16,1>)  [unwired: 1 in]
        n2181 = property on="Trap Pos FB SP" class="DigNum (strict)"("Val(Sgnl)"=w3271) -> ()  [unwired: 2 in, 2 out]
      }
      event "inject shunt": Value Change {
        n2182 = event-data() -> ()  [unwired: 7 out]
        n2183 = call "hamilton_controller.vi"("Open?"="inject shunt", "valve"=enum16{"A", "B", "C", "D", "ALL"}."D", "action"=T42."MOVE VALVE") -> ("error out"=w3305:errorcluster)  [unwired: 7 in, 1 out]
      }
      event "Trap 3 (ON/OFF)", "T3 Y (V)", "T3 X (V)": Value Change {
        n2184 = event-data() -> ()  [unwired: 7 out]
        n2185 = case shown="False" "Trap 3 (ON/OFF)" {
          tunnel: [5.0 0.0] -> w3310
          frame False {
          }
          frame True {
          }
        }
        n2186 = Multiply(x="T3 X (V)", y=32767.0) -> (x*y=w3326:dbl)
        n2187 = Multiply(x="T3 Y (V)", y=32767.0) -> (x*y=w3323:dbl)
        n2188 = Divide(x=w3326, y=10.0) -> (x/y=w3327:dbl)
        n2189 = Divide(x=w3323, y=10.0) -> (x/y=w3322:dbl)
        n2190 = To Unsigned Word Integer(number=w3327) -> (unsigned 16bit integer=w3316:u16)
        n2191 = To Unsigned Word Integer(number=w3322) -> (unsigned 16bit integer=w3317:u16)
        n2192 = Multiply(x=w3310, y=32767.0) -> (x*y=w3313:dbl)
        n2193 = Divide(x=w3313, y=10.0) -> (x/y=w3312:dbl)
        n2194 = To Unsigned Word Integer(number=w3312) -> (unsigned 16bit integer=w3309:u16)
        n2195 = xnode "Read/Write Control"("FPGA VI Reference In"=w3318, "Piezo Trap X (AO5)"=w3316, "Piezo Trap Y (AO4)"=w3317, "Piezo Trap ON/Off (AO3)"=w3309) -> ()  [unwired: 1 in, 2 out]
      }
      event "Cursor control.X", "Cursor control.Y": Value Change {
        # "If turning cursor control off, update the piezo controls"
        n2196 = event-data() -> ()  [unwired: 7 out]
        n2197 = xnode "Read/Write Control"("FPGA VI Reference In"=w3337) -> ("Piezo X out"=w3335:u16, "Piezo Y out"=w3331:u16)  [unwired: 1 in, 2 out]
        n2198 = local read "Cursor control"() -> (w3336:cluster{"X":bool, "Y":bool})
        n2199 = Unbundle By Name(w3336) -> ("X"=w3334:bool, "Y"=w3333:bool)
        n2200 = And(x=w3334, y=w3333) -> (x .and. y?=w3332:bool)
        n2201 = case shown="True" w3332 {
          tunnel: w3335 -> [w3342 _]
          tunnel: w3331 -> [w3340 _]
          frame False {
            w3339 = 3276.7
            n2202 = Divide(x=w3342, y=w3339) -> (x/y=w3341:dbl)
            n2203 = Divide(x=w3340, y=w3339) -> (x/y=w3338:dbl)
            n2204 = property on="T3 X (V)" class="DigNum (strict)"("Val(Sgnl)"=w3341) -> ()  [unwired: 2 in, 2 out]
            n2205 = property on="T3 Y (V)" class="DigNum (strict)"("Val(Sgnl)"=w3338) -> ()  [unwired: 2 in, 2 out]
          }
          frame True {
          }
        }
      }
    }
    "error out 2" <- w1717
    n2206 = node-c288() -> ()  [unwired: 2 out]
  }
  n2207 = node-c288() -> (w67:T37)  [unwired: 4 out]
  n2208 = timed-loop "Mouse control: trap position (AOM deflection), set confocal spot from image" {
    tunnel: [w3343] -> w72
    timing: w67 -> [_]
    timing-out: [_] -> w66
    tunnel: w24 -> [w3344]
    stop <- w3343 stop-if-true
    n2209 = node-c288() -> ()  [unwired: 2 out]
    n2210 = event shown="[0] \"Pane\": Mouse Down" {
      selector: _ -> [_ _ _ _]
      dyn-events: _ -> [_ _ _ _]
      timeout: _ -> [_ _ _ _]
      tunnel: w3344 -> [w3347 _ _ _]
      tunnel: [_ _ TRUE _] -> w3343
      event Mouse Down {
        n2211 = event-data() -> ("Time"=w3349:u32, "Coords"=w3348:T12, "Button"=w3350:u16)  [unwired: 6 out]
        n2212 = case shown="1" w3350 {
          tunnel: w3349 -> [_ _ w3456]
          tunnel: w3348 -> [_ w3387 w3454]
          tunnel: w3347 -> [_ _ w3450]
          frame 0, Default {
          }
          frame 1 {
            n2213 = property on="APD 2"() -> ("Displayed Image Size"=w3356)  [unwired: 2 in, 2 out]
            n2214 = property on="APD 1"() -> ("Displayed Image Size"=w3384)  [unwired: 2 in, 2 out]
            n2215 = property on="Detection Laser X"() -> ("Displayed Image Size"=w3385)  [unwired: 2 in, 2 out]
            n2216 = property on="Detection Laser Y"() -> ("Displayed Image Size"=w3381)  [unwired: 2 in, 2 out]
